vi "SWERVE_DRIVE_MODULE_ACT.vi"(6 "Pass_Through_Time":dbl=-1.0 format="%33.4f", 8 "SwervePosInDeadband":bool=TRUE, 9 "Swerve Sense":T1={"Speed"=0.0, "Angle"={"VALUE"=0.0, "COS"=1.0, "SIN"=0.0}} {"Angle"."SIN" format="%13.4f"; "Angle"."COS" format="%13.4f"; "Angle"."VALUE" format="%13.4f"}, 10 "Swerve Dmd":T1={"Speed"=0.0, "Angle"={"VALUE"=0.0, "COS"=1.0, "SIN"=0.0}} {"Angle"."SIN" format="%13.4f"; "Angle"."COS" format="%13.4f"; "Angle"."VALUE" format="%13.4f"}, 11 "Swerve Module TypDef":T3) -> (0 "SwerveOnTarget":bool, 1 "SwervePosError":dbl, 2 "Swerve Motor Dmd":dbl, 3 "Wheel Motor Dmd":dbl, 4 "WheelSpeedErr":dbl)   [LabVIEW 2019]
uses:
  SWERVE_DRIVE_MODULE_TYPDEF.ctl
  <vilib>/Rock Robotics/WPI/MotorControl/WPI_MotorControlDeviceRef.ctl
  <vilib>/Rock Robotics/WPI/MotorControl/WPI_MotorControlType.ctl
  <vilib>/Rock Robotics/SystemInterfaces/DIO/FPGA_DIOPWMChannel.ctl
  <vilib>/Rock Robotics/WPI/PWM/WPI_PWMDeadband.ctl
  <vilib>/Rock Robotics/SystemInterfaces/DIO/FPGA_DIOChannel.ctl
  <vilib>/Rock Robotics/WPI/Encoder/WPI_EncoderDevRef.ctl
  <vilib>/Rock Robotics/SystemInterfaces/Encoder/FPGA_EncoderIdx.ctl
  <vilib>/Rock Robotics/SystemInterfaces/Counter/FPGA_CounterCtrSystemIndex.ctl
  <vilib>/Rock Robotics/WPI/Encoder/WPI_EncoderType.ctl
  <vilib>/Rock Robotics/WPI/ThirdParty/JAS_Junk/TrajLib/TypeDef/SWERVE_DRIVE_MODULE_STATE.ctl
  <vilib>/Rock Robotics/WPI/ThirdParty/JAS_Junk/TrajLib/TypeDef/ROTATION2D.ctl
  <vilib>/Rock Robotics/WPI/ThirdParty/JAS_Junk/TrajLib/TypeDef/X_Y_PAIR.ctl
  <vilib>/Rock Robotics/WPI/ThirdParty/JAS_Junk/TrajLib/MathUtil_InputModulus.vi
  <vilib>/Rock Robotics/WPI/ThirdParty/JAS_Junk/TrajLib/Rotation2d_Minus.vi
  <vilib>/Rock Robotics/WPI/ThirdParty/JAS_Junk/TrajLib/Rotation2d_GetRadians.vi
  <vilib>/Rock Robotics/WPI/ThirdParty/JAS_Junk/TrajLib/SwerveModuleState_New.vi
  <vilib>/Rock Robotics/WPI/ThirdParty/JAS_Junk/TrajLib/Rotation2d_RotateBy.vi
  <vilib>/Rock Robotics/WPI/ThirdParty/JAS_Junk/TrajLib/Rotation2d_CreateAngle.vi
  <vilib>/Rock Robotics/WPI/ThirdParty/JAS_Junk/TrajLib/VI/FunctionGenerator_New.vi
  <vilib>/Rock Robotics/WPI/ThirdParty/JAS_Junk/TrajLib/VI/FunctionGenerator_Calculate.vi
  <vilib>/Rock Robotics/WPI/ThirdParty/JAS_Junk/TrajLib/PIDController_AtSetpoint.vi
  <vilib>/Rock Robotics/WPI/ThirdParty/JAS_Junk/TrajLib/PIDController_SetPIDF.vi
  <vilib>/Rock Robotics/WPI/ThirdParty/JAS_Junk/TrajLib/PIDController_SetDerivativeFilter.vi
  <vilib>/Rock Robotics/WPI/ThirdParty/JAS_Junk/TrajLib/PIDController_SetIntegratorRange.vi
  <vilib>/Rock Robotics/WPI/ThirdParty/JAS_Junk/TrajLib/PIDController_SetTolerancePandV.vi
  <vilib>/Rock Robotics/WPI/ThirdParty/JAS_Junk/TrajLib/PIDController_DisableContinousInput.vi
  <vilib>/Rock Robotics/WPI/ThirdParty/JAS_Junk/TrajLib/PIDController_EnableContinousInput.vi
  <vilib>/Rock Robotics/WPI/ThirdParty/JAS_Junk/TrajLib/PIDController_Reset.vi
  <vilib>/Rock Robotics/WPI/ThirdParty/JAS_Junk/TrajLib/PIDController_New.vi
  <vilib>/Rock Robotics/WPI/ThirdParty/JAS_Junk/TrajLib/PIDController_SetOutputLimits.vi
  <vilib>/Rock Robotics/WPI/ThirdParty/JAS_Junk/TrajLib/SlewRateLimiter_New.vi
  <vilib>/Rock Robotics/WPI/ThirdParty/JAS_Junk/TrajLib/SlewRateLimiter_Reset.vi
  <vilib>/Rock Robotics/WPI/ThirdParty/JAS_Junk/TrajLib/SlewRateLimiter_Calculate.vi
  <vilib>/Rock Robotics/WPI/ThirdParty/JAS_Junk/TrajLib/SlewRateLimiter_SetRate.vi
  <vilib>/Rock Robotics/WPI/ThirdParty/JAS_Junk/TrajLib/Rotation2d_UnaryMinus.vi
  <vilib>/Rock Robotics/WPI/ThirdParty/JAS_Junk/TrajLib/Rotation2d_CreateXY.vi
  <vilib>/Rock Robotics/WPI/ThirdParty/JAS_Junk/TrajLib/PIDController_NewPeriod.vi
  <vilib>/Rock Robotics/WPI/ThirdParty/JAS_Junk/TrajLib/Util_CalcDist.vi
  <vilib>/Rock Robotics/SystemInterfaces/NetworkCommunication/NetComm_UsageReport_report.vi
  <vilib>/gmath/interp.llb/Search Ordered Table.vi
  <vilib>/Rock Robotics/WPI/ThirdParty/JAS_Junk/TrajLib/Util_LibraryGlobals.vi
  <vilib>/Rock Robotics/WPI/ThirdParty/JAS_Junk/TrajLib/PIDController_AdvCalculate_FF_Sp_Pv.vi
  <vilib>/Rock Robotics/WPI/ThirdParty/JAS_Junk/TrajLib/Trajectory_Library.lvlib
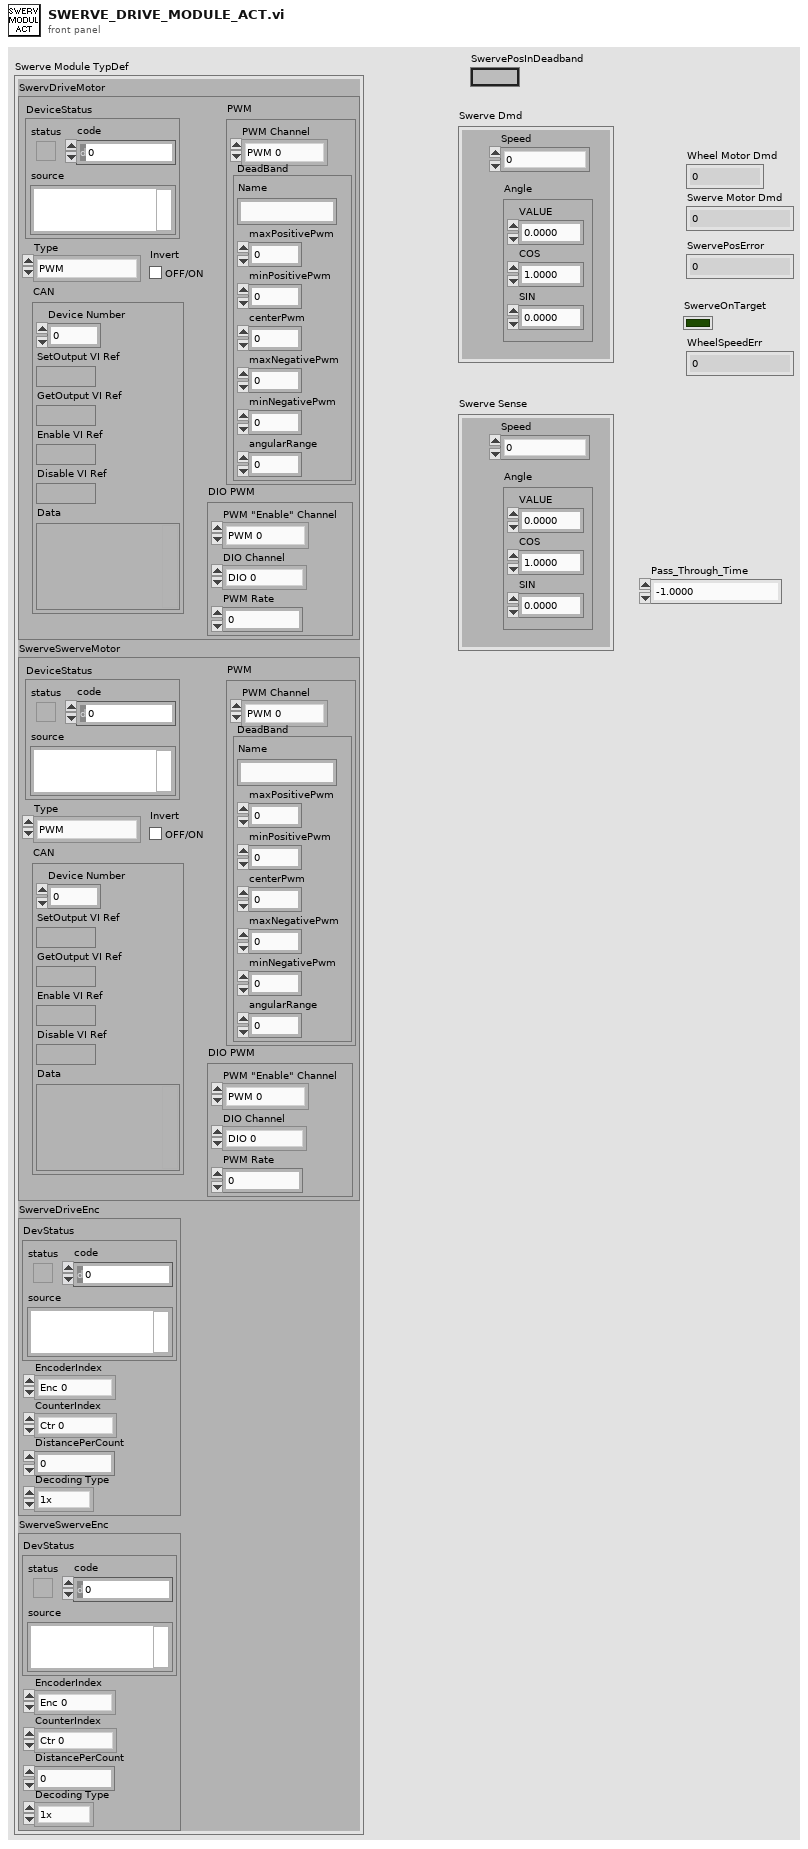
[diagram p1: front panel]
types:
  T1 = typedef "Trajectory_Library.lvlib/SWERVE_DRIVE_MODULE_STATE.ctl" = cluster{"Speed":dbl, "Angle":T2}
  T2 = typedef "Trajectory_Library.lvlib/ROTATION2D.ctl" = cluster{"VALUE":dbl, "COS":dbl, "SIN":dbl}
  T3 = typedef "SWERVE_DRIVE_MODULE_TYPDEF.ctl" = cluster{"SwervDriveMotor":T4, "SwerveSwerveMotor":T4, "SwerveDriveEnc":T9, "SwerveSwerveEnc":T9}
  T4 = typedef "WPI_MotorControlDeviceRef.ctl" = cluster{"DeviceStatus":errorcluster, "Type":T5, "PWM":cluster{"PWM Channel":T6, "DeadBand":T7}, "CAN":cluster{"Device Number":u8, "SetOutput VI Ref":variant, "GetOutput VI Ref":variant, "Enable VI Ref":variant, "Disable VI Ref":variant, "Data":variant}, "Invert":bool, "DIO PWM":cluster{"PWM \"Enable\" Channel":T6, "DIOChannel":T8, "PWM Rate":dbl}}
  T5 = typedef "WPI_MotorControlType.ctl" = enum16{"PWM", "CAN", "DIO PWM"}
  T6 = typedef "FPGA_DIOPWMChannel.ctl" = enum8{"PWM 0", "PWM 1", "PWM 2", "PWM 3", "PWM 4", "PWM 5", "PWM 6", "PWM 7", "PWM 8", "PWM 9", "PWM MXP 0", "PWM MXP 1", "PWM MXP 2", "PWM MXP 3", "PWM MXP 4", "PWM MXP 5", "PWM MXP 6", "PWM MXP 7", "PWM MXP 8", "PWM MXP 9", "Invalid"}
  T7 = typedef "WPI_PWMDeadband.ctl" = cluster{"Name":string, "maxPositivePwm":i32, "minPositivePwm":i32, "centerPwm":i32, "maxNegativePwm":i32, "minNegativePwm":i32, "angularRange":u16}
  T8 = typedef "FPGA_DIOChannel.ctl" = enum8{"DIO 0", "DIO 1", "DIO 2", "DIO 3", "DIO 4", "DIO 5", "DIO 6", "DIO 7", "DIO 8", "DIO 9", "DIO MXP 0", "DIO MXP 1", "DIO MXP 2", "DIO MXP 3", "DIO MXP 4", "DIO MXP 5", "DIO MXP 6", "DIO MXP 7", "DIO MXP 8", "DIO MXP 9", "DIO MXP 10", "DIO MXP 11", "DIO MXP 12", "DIO MXP 13", "DIO MXP 14", "DIO MXP 15", "SPI Port CS1", "SPI Port CS2", "SPI Port CS3", "SPI Port MISO", "SPI Port MOSI", "Invalid"}
  T9 = typedef "WPI_EncoderDevRef.ctl" = cluster{"DevStatus":errorcluster, "EncoderIndex":T10, "CounterIndex":T11, "DistancePerCount":dbl, "Decoding Type":T12}
  T10 = typedef "FPGA_EncoderIdx.ctl" = enum8{"Enc 0", "Enc 1", "Enc 2", "Enc 3", "Enc 4", "Enc 5", "Enc 6", "Enc 7", "Invalid"}
  T11 = typedef "FPGA_CounterCtrSystemIndex.ctl" = enum8{"Ctr 0", "Ctr 1", "Ctr 2", "Ctr 3", "Ctr 4", "Ctr 5", "Ctr 6", "Ctr 7", "Invalid"}
  T12 = typedef "WPI_EncoderType.ctl" = enum16{"1x", "2x", "4x"}
  T13 = typedef "Trajectory_Library.lvlib/X_Y_PAIR.ctl" = cluster{"X":dbl, "Y":dbl}
  T14 = typedef "Trajectory_Library.lvlib/PID_ADV_LIMITS.ctl" = cluster{"MaxInput":dbl, "MinInput":dbl, "Continuous":bool, "MaxOutput":dbl, "MinOutput":dbl}
  T15 = typedef "Trajectory_Library.lvlib/PID_ADV_TUNING.ctl" = cluster{"Kf":dbl, "Kp":dbl, "Ki":dbl, "Kd":dbl, "MaximumIntegral":dbl, "MinimumIntegral":dbl, "Filter Derivative":bool}
  T16 = typedef "Trajectory_Library.lvlib/PID_CONTROLLER.ctl" = cluster{"Kp":dbl, "Ki":dbl, "Kd":dbl, "Period":dbl, "Max_Integral":dbl, "Min_Integral":dbl, "Max_Input":dbl, "Min_Input":dbl, "Continuous":bool, "PositionError":dbl, "VelocityError":dbl, "PrevError":dbl, "TotalError":dbl, "PositionTolerance":dbl, "VelocityTolerance":dbl, "SetPoint":dbl, "Kf":dbl, "Prev_Deriv":dbl, "Prev_Deriv 2":dbl, "DerivativeFilter":bool, "Min_Output":dbl, "Max_Output":dbl, "Prev_F_P":dbl, "Prev_F_P_2":dbl, "AntiWindupActive":bool, "Measurement":dbl}
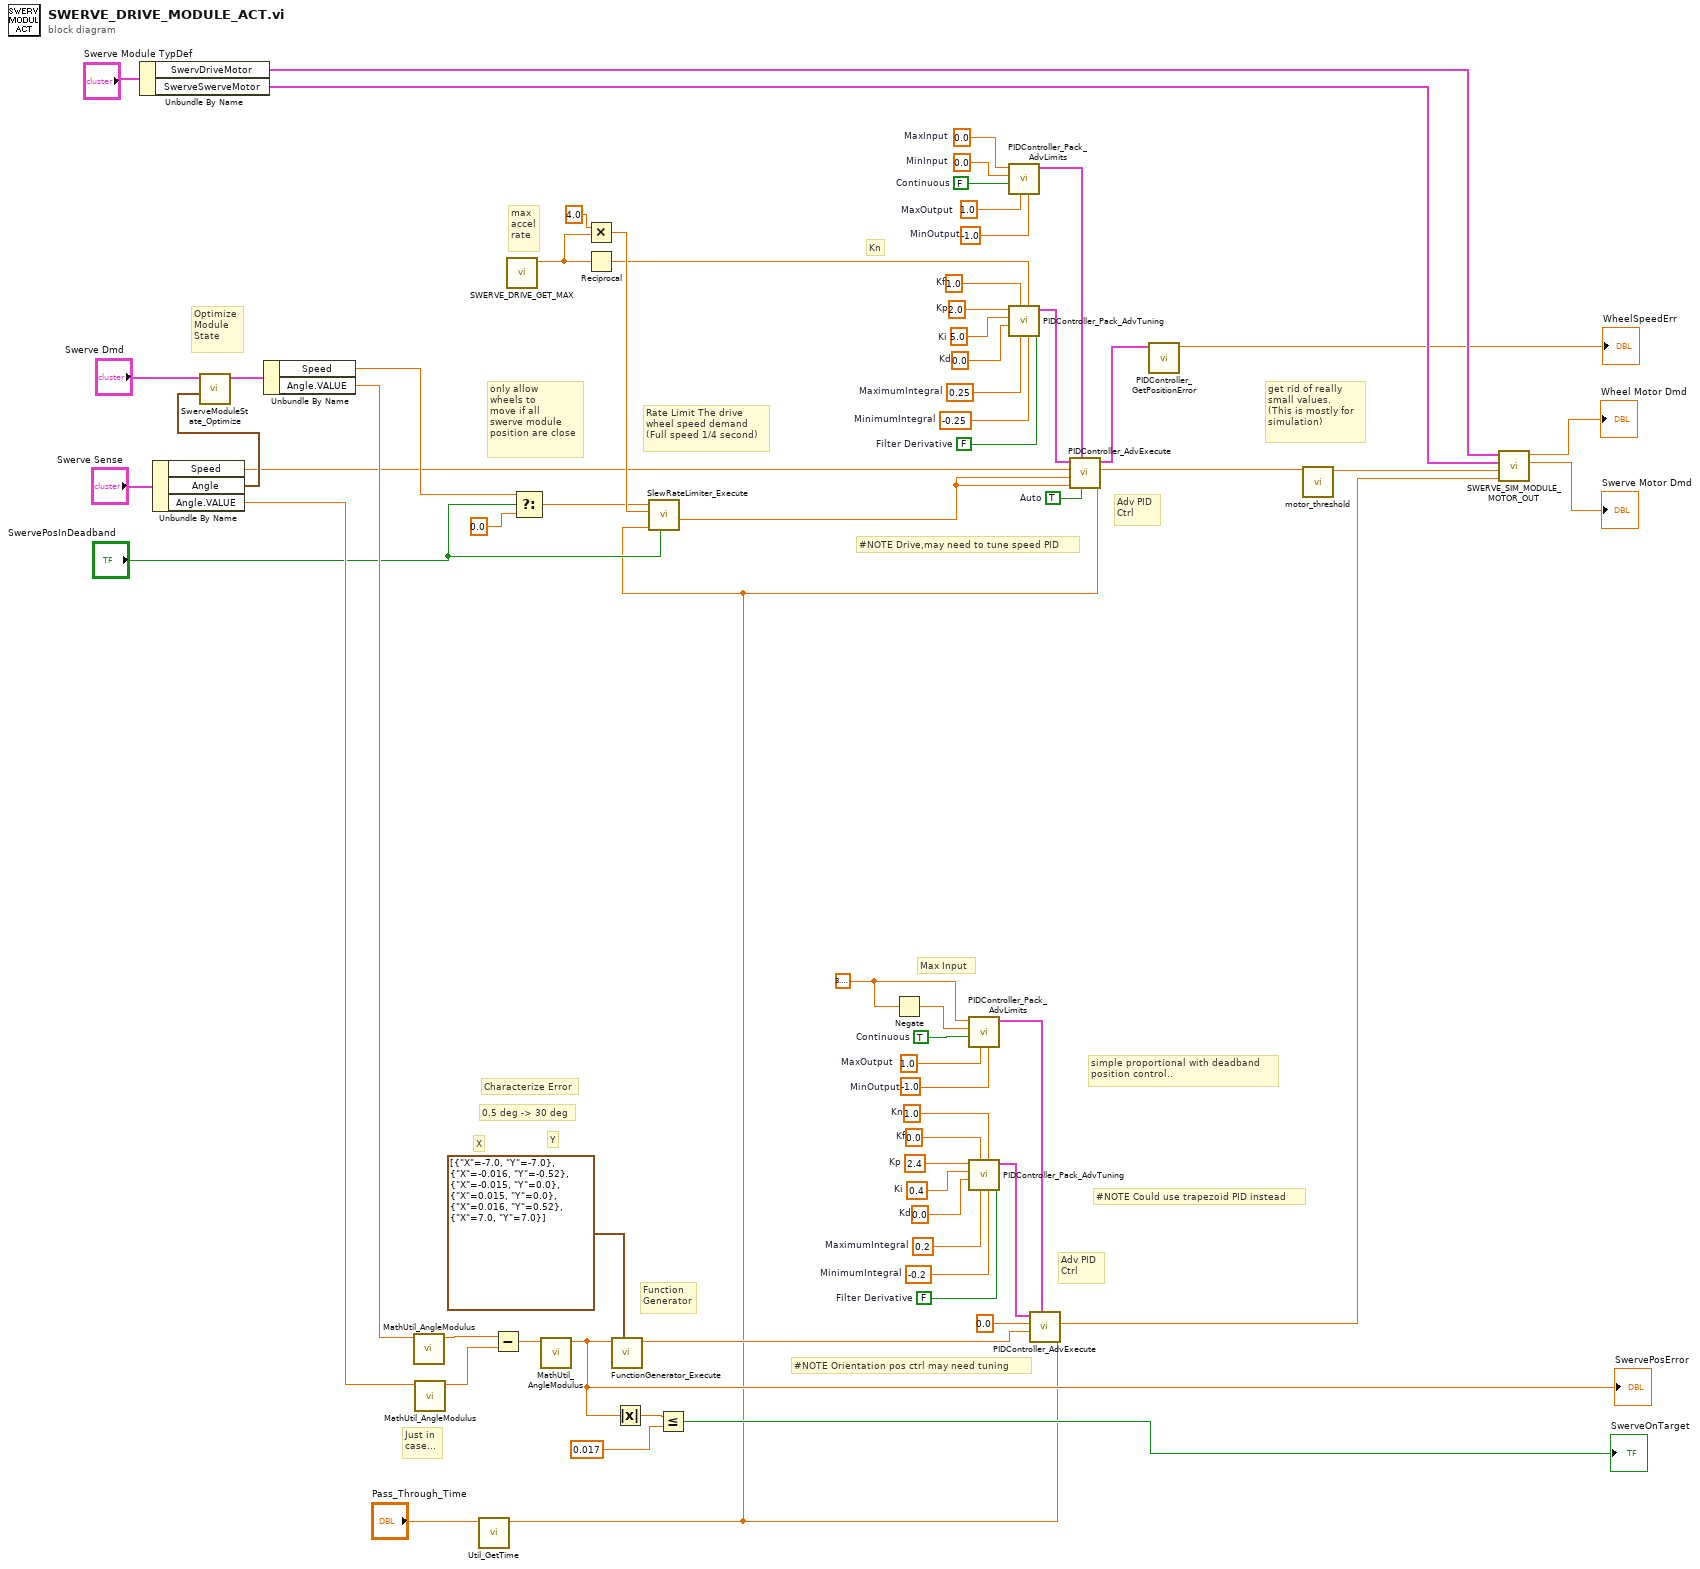
[diagram p0: block diagram]
diagram:
  w6 = TRUE  # Auto
  w22 = 2.0  # Kp
  w21 = 5.0  # Ki
  w20 = 0.0  # Kd
  w19 = 1.0  # Kf
  w18 = 0.25  # MaximumIntegral
  w17 = -0.25  # MinimumIntegral
  w16 = FALSE  # Filter Derivative
  w14 = 0.0  # MinInput
  w13 = FALSE  # Continuous
  w12 = 1.0  # MaxOutput
  w15 = -1.0  # MinOutput
  w11 = 0.0  # MaxInput
  w39 = 1.0  # MaxOutput
  w40 = -1.0  # MinOutput
  w44 = 3.141592653589793
  w55 = 1.0  # Kn
  w54 = 2.4  # Kp
  w53 = 0.4  # Ki
  w52 = 0.0  # Kd
  w51 = 0.0  # Kf
  w50 = 0.2  # MaximumIntegral
  w49 = -0.2  # MinimumIntegral
  w48 = FALSE  # Filter Derivative
  w47 = TRUE  # Continuous
  # "Optimize\nModule\nState"
  # "Kn"
  # "Adv PID\nCtrl"
  # "Rate Limit The drive\nwheel speed demand\n(Full speed 1/4 second)"
  # "Just in \ncase..."
  # "#NOTE Could use trapezoid PID instead"
  # "Characterize Error"
  # "Max Input"
  # "Adv PID\nCtrl"
  # "0.5 deg -> 30 deg"
  # "Function\nGenerator"
  # "Y"
  # "X"
  # "#NOTE Orientation pos ctrl may need tuning"
  # "only allow\nwheels to \nmove if all \nswerve module \nposition are close"
  # "#NOTE Drive,may need to tune speed PID"
  # "simple proportional with deadband\nposition control.."
  # "get rid of really\nsmall values.\n(This is mostly for \nsimulation)"
  # "max\naccel\nrate"
  n1 = Unbundle By Name("Swerve Module TypDef") -> ("SwervDriveMotor"=w62:T4, "SwerveSwerveMotor"=w64:T4)
  n2 = Unbundle By Name("Swerve Sense") -> ("Speed"=w7:dbl, "Angle"=w26:T2, "Angle.VALUE"=w27:dbl)
  n3 = call <vilib>:"SwerveModuleState_Optimize.vi"("CurrentAngle"=w26, "Desired State"="Swerve Dmd") -> ("out SWERVE_DRIVE_MODULE_STATE"=w25:T1)  [unwired: 9 in]
  n4 = Unbundle By Name(w25) -> ("Speed"=w24:dbl, "Angle.VALUE"=w33:dbl)
  n5 = call <vilib>:"MathUtil_AngleModulus.vi"("InputAngle"=w33) -> ("ModulsAngle"=w32:dbl)  [unwired: 10 in]
  n6 = call <vilib>:"MathUtil_AngleModulus.vi"("InputAngle"=w27) -> ("ModulsAngle"=w31:dbl)  [unwired: 10 in]
  n7 = call <vilib>:"Util_GetTime.vi"("Pass_Through_Time"="Pass_Through_Time") -> ("FPGA_Time_Seconds"=w2:dbl)  [unwired: 9 in, 1 out]
  n8 = Subtract(x=w32, y=w31) -> (x-y=w34:dbl)
  n9 = call "SWERVE_DRIVE_GET_MAX.vi"() -> ("Max Wheel Vel (Meter/Sec)"=w66:dbl)  [unwired: 10 in, 1 out]
  n10 = Select(t=w24, s="SwervePosInDeadband", f=0.0) -> (s? t:f=w58:dbl)
  n11 = call <vilib>:"MathUtil_AngleModulus.vi"("InputAngle"=w34) -> ("ModulsAngle"=w30:dbl)  [unwired: 10 in]
  "SwervePosError" <- w30
  n12 = Multiply(x=4.0, y=w66) -> (x*y=w59:dbl)
  n13 = Reciprocal(x=w66) -> (1/x=w8:dbl)
  n14 = call <vilib>:"FunctionGenerator_Execute.vi"("X Y Pairs"=T13[] [{"X"=-7.0, "Y"=-7.0}, {"X"=-0.016, "Y"=-0.52}, {"X"=-0.015, "Y"=0.0}, {"X"=0.015, "Y"=0.0}, {"X"=0.016, "Y"=0.52}, {"X"=7.0, "Y"=7.0}], "Input Value"=w30) -> ("Output Value"=w41:dbl)  [unwired: 9 in]
  n15 = Absolute Value(x=w30) -> (abs(x)=w38:dbl)
  n16 = call <vilib>:"SlewRateLimiter_Execute.vi"("Enable"="SwervePosInDeadband", "Time"=w2, "PositiveRate"=w59, "Input"=w58) -> ("Output"=w1:dbl)  [unwired: 6 in, 1 out]
  n17 = Less Or Equal?(x=w38, y=0.017 ("ErrDeadband")) -> (x <= y?=→"SwerveOnTarget":bool)
  n18 = Negate(x=w44) -> (-x=w43:dbl)
  n19 = call <vilib>:"PIDController_Pack_AdvLimits.vi"("MinOutput"=w40, "MaxOutput"=w39, "Continuous"=w47, "MinInput"=w43, "MaxInput"=w44) -> ("Adv PID Limits"=w45:T14)  [unwired: 6 in]
  n20 = call <vilib>:"PIDController_Pack_AdvTuning.vi"("Filter Derivative"=w48, "MinimumIntegral"=w49, "Kn"=w55, "MaximumIntegral"=w50, "Kf"=w51, "Kd"=w52, "Ki"=w53, "Kp"=w54) -> ("Adv PID Tuning"=w46:T15)  [unwired: 3 in]
  n21 = call <vilib>:"PIDController_Pack_AdvLimits.vi"("MinOutput"=w15, "MaxOutput"=w12, "Continuous"=w13, "MinInput"=w14, "MaxInput"=w11) -> ("Adv PID Limits"=w9:T14)  [unwired: 6 in]
  n22 = call <vilib>:"PIDController_Pack_AdvTuning.vi"("Filter Derivative"=w16, "MinimumIntegral"=w17, "Kn"=w8, "MaximumIntegral"=w18, "Kf"=w19, "Kd"=w20, "Ki"=w21, "Kp"=w22) -> ("Adv PID Tuning"=w10:T15)  [unwired: 3 in]
  n23 = call <vilib>:"PIDController_AdvExecute.vi"("Time"=w2, "Adv PID Limits"=w45, "SP-SetPoint"=w41, "PV-Measurement"=0.0, "Adv PID Tuning"=w46) -> ("CO-ControlOutput"=w35:dbl)  [unwired: 4 in, 2 out]
  n24 = call <vilib>:"PIDController_AdvExecute.vi"("Time"=w2, "Auto"=w6, "Adv PID Limits"=w9, "FF-FeedForward"=w1, "SP-SetPoint"=w1, "PV-Measurement"=w7, "Adv PID Tuning"=w10) -> ("CO-ControlOutput"=w5:dbl, "out PID_CONTROLLER"=w4:T16)  [unwired: 2 in, 1 out]
  n25 = call <vilib>:"PIDController_GetPositionError.vi"("in PID_CONTROLLER"=w4) -> ("PositionError"=→"WheelSpeedErr":dbl)  [unwired: 10 in]
  n26 = call "motor_threshold.vi"("motor in"=w5) -> ("motor out"=w63:dbl)  [unwired: 10 in]
  n27 = call "SWERVE_SIM_MODULE_MOTOR_OUT.vi"("SwerveOutput"=w35, "DriveOutput"=w63, "SwerveSwerveMotor"=w64, "SwervDriveMotor"=w62) -> ("SwerveMotorDmd"=→"Swerve Motor Dmd":dbl, "WheelMotorDmd"=→"Wheel Motor Dmd":dbl)  [unwired: 6 in]
